vi "process_nodes.vi"(0 "embed_nodes in":refnum<class "embed_nodes.lvclass">, 5 "nodes":refnum<class "data_node.lvclass">[](array[class]), 11 "error in (no error)":errorcluster) -> (4 "embed_nodes out":refnum<class "embed_nodes.lvclass">, 6 "nodes":refnum<class "data_node.lvclass">[](array[class]), 15 "error out":errorcluster)   [LabVIEW 2020, in "embed_nodes.lvclass"]
uses:
  embed_nodes.lvclass
  data/data_node/data_node.lvclass
  embed_nodes.lvclass/embed_nodes.ctl
  models/message_text/message_text.lvclass
  D:/Personal/LabVIEW LLMs/src/models/abstract_message_base/abstract_message_base.lvclass
  models/message_vectors/message_vectors.lvclass
  models/abstract_llm_embedding/abstract_llm_embedding.lvclass
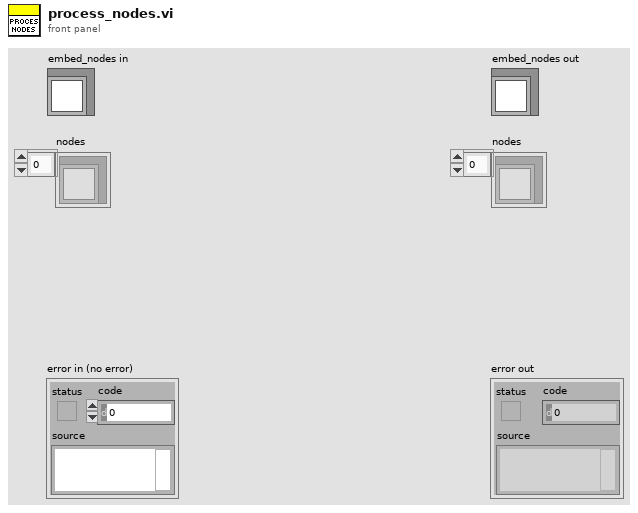
[diagram p1: front panel]
types:
  T1 = typedef "message_vectors.lvclass/embedding.ctl" = cluster{"index":u32, "Vectors":dbl[]}
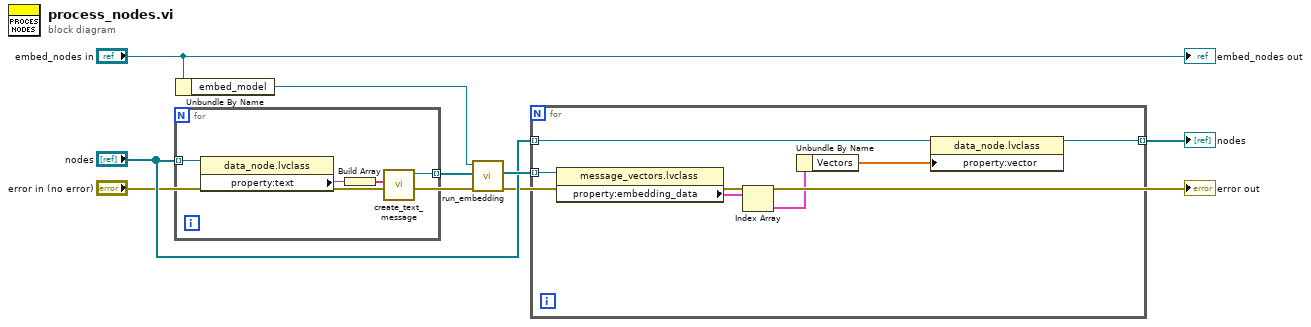
[diagram p0: block diagram]
diagram:
  n1 = for {
    tunnel: "nodes" -> [w12] mode=indexing
    tunnel: [w9] -> w7 mode=indexing
    n2 = property class="data_node.lvclass"(reference=w12) -> ("property:text"=w11:string)  [unwired: 1 in, 2 out]
    n3 = Build Array(w11) -> (w10:string[])
    n4 = call "create_text_message.vi"("content"=w10) -> ("message_text out"=w9:refnum<class "message_text.lvclass">)  [unwired: 9 in, 1 out]
  }
  n5 = Unbundle By Name("embed_nodes in") -> ("embed_model"=w8:refnum<class "abstract_llm_base.lvclass">)
  n6 = call "run_embedding.vi"("error in (no error)"="error in (no error)", "Messages"=w7, "abstract_llm_embedding in"=w8) -> ("error out"=→"error out":errorcluster, "Response"=w6:refnum<class "message_vectors.lvclass">[])  [unwired: 6 in, 1 out]
  n7 = for {
    tunnel: w6 -> [w18] mode=indexing
    tunnel: "nodes" -> [w15] mode=indexing
    tunnel: [w13] -> w1 mode=indexing
    n8 = property class="message_vectors.lvclass"(reference=w18) -> ("property:embedding_data"=w17:T1[])  [unwired: 1 in, 2 out]
    n9 = Index Array(array=w17) -> (element=w16:T1)  [unwired: 1 in]
    n10 = Unbundle By Name(w16) -> ("Vectors"=w14:dbl[])
    n11 = property class="data_node.lvclass"(reference=w15, "property:vector"=w14) -> (reference out=w13:refnum<class "data_node.lvclass">)  [unwired: 1 in, 1 out]
  }
  "nodes" <- w1
  "embed_nodes out" <- "embed_nodes in"
